vi "CA.vi"(0 "OUTPUT VARS":refnum<vi>, 1 "INPUT VARS":refnum<vi>, 2 "States":refnum<vi>, 3 "AlgStates":refnum<vi>, 4 "Processes":refnum<vi>, 5 "INP":refnum<vi>, 6 "PORTS":refnum<vi>) -> ()   [LabVIEW 2010]
panel:
  out "Здачения 2":string[](array[string])
  out "Типы 2":string[](array[string])
  out "Output:":string[](array[string])
  out "Value:":string[](array[string])
  out "Type:":string[](array[string])
  out "Input:":string[](array[string])
  out "Cluster":T1
  in  "algOutputMsgs":refnum<vi>
  in  "CA2GUI":refnum<vi>
  out "Output messages":T2(array[cluster])
  in  "OUTP":refnum<vi>
  out "Value":T3
  out "States of processes:":string[][](table)
  in  "OUT Ports Array":cluster{"Port":string, "Value":bool[]}[](array[cluster])
  in  "INP Ports Array":cluster{"Port\nPort":string, "Value":bool[]}[](array[cluster])
  # "Control algorithm"
  # "Global variables"
  # "Input ports values"
  # "Output ports values"
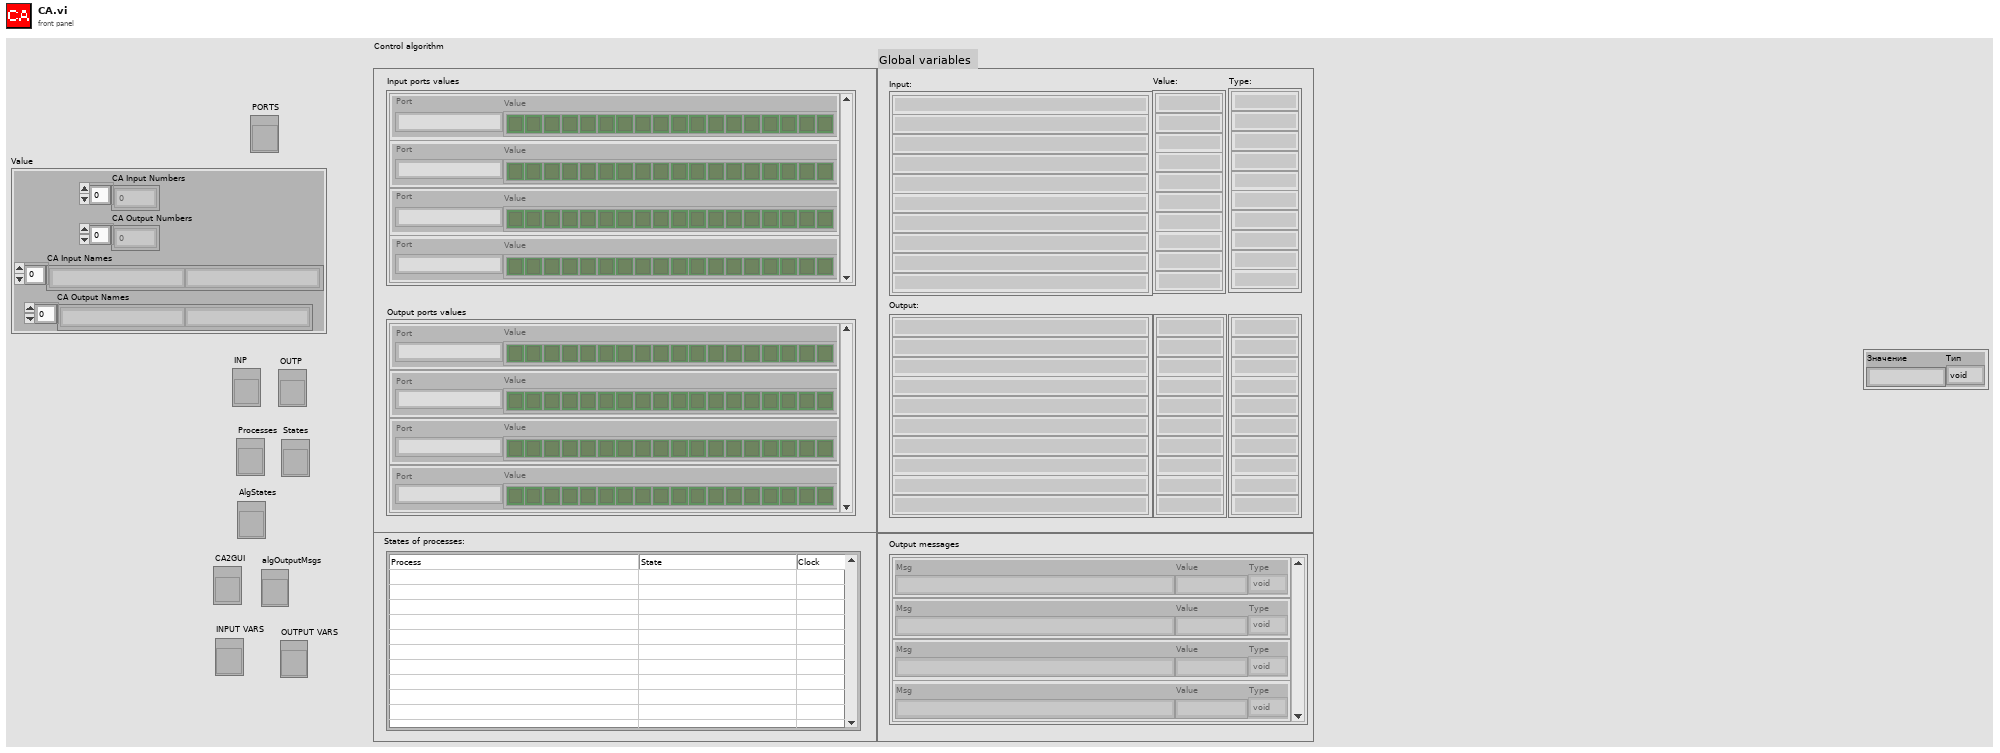
[diagram p1: front panel]
types:
  T1 = cluster{"Значение":string, "Тип":enum16{"void", "byte", "int", "float"}}
  T2 = cluster{"Msg":string, "Value":string, "Type":enum16{"void", "byte", "int", "float"}}[]
  T3 = cluster{"CA Input Numbers":i32[], "CA Output Numbers ":i32[], "CA Input Names":string[], "CA Output Names ":string[]}
  T4 = cluster{"Сообщение":string, "Значение":string, "Тип":enum16{"void", "byte", "int", "float"}}
  T5 = cluster{"Input varables names":string[], "Input varables type":string[], "Input varables ports":i32[], "Input varables bytes":i32[]}
  T6 = cluster{"Output varables names":string[], "Output varables type":string[], "Output varables ports":i32[], "Output varables bytes":i32[]}
  T7 = cluster{"Сообщение":string, "Значение":string, "Тип":enum16{"void", "byte", "int", "float"}}[]
  T8 = cluster{"MSG":i16, "param":i32, "Type":enum16{"void", "byte", "int", "float"}}[]
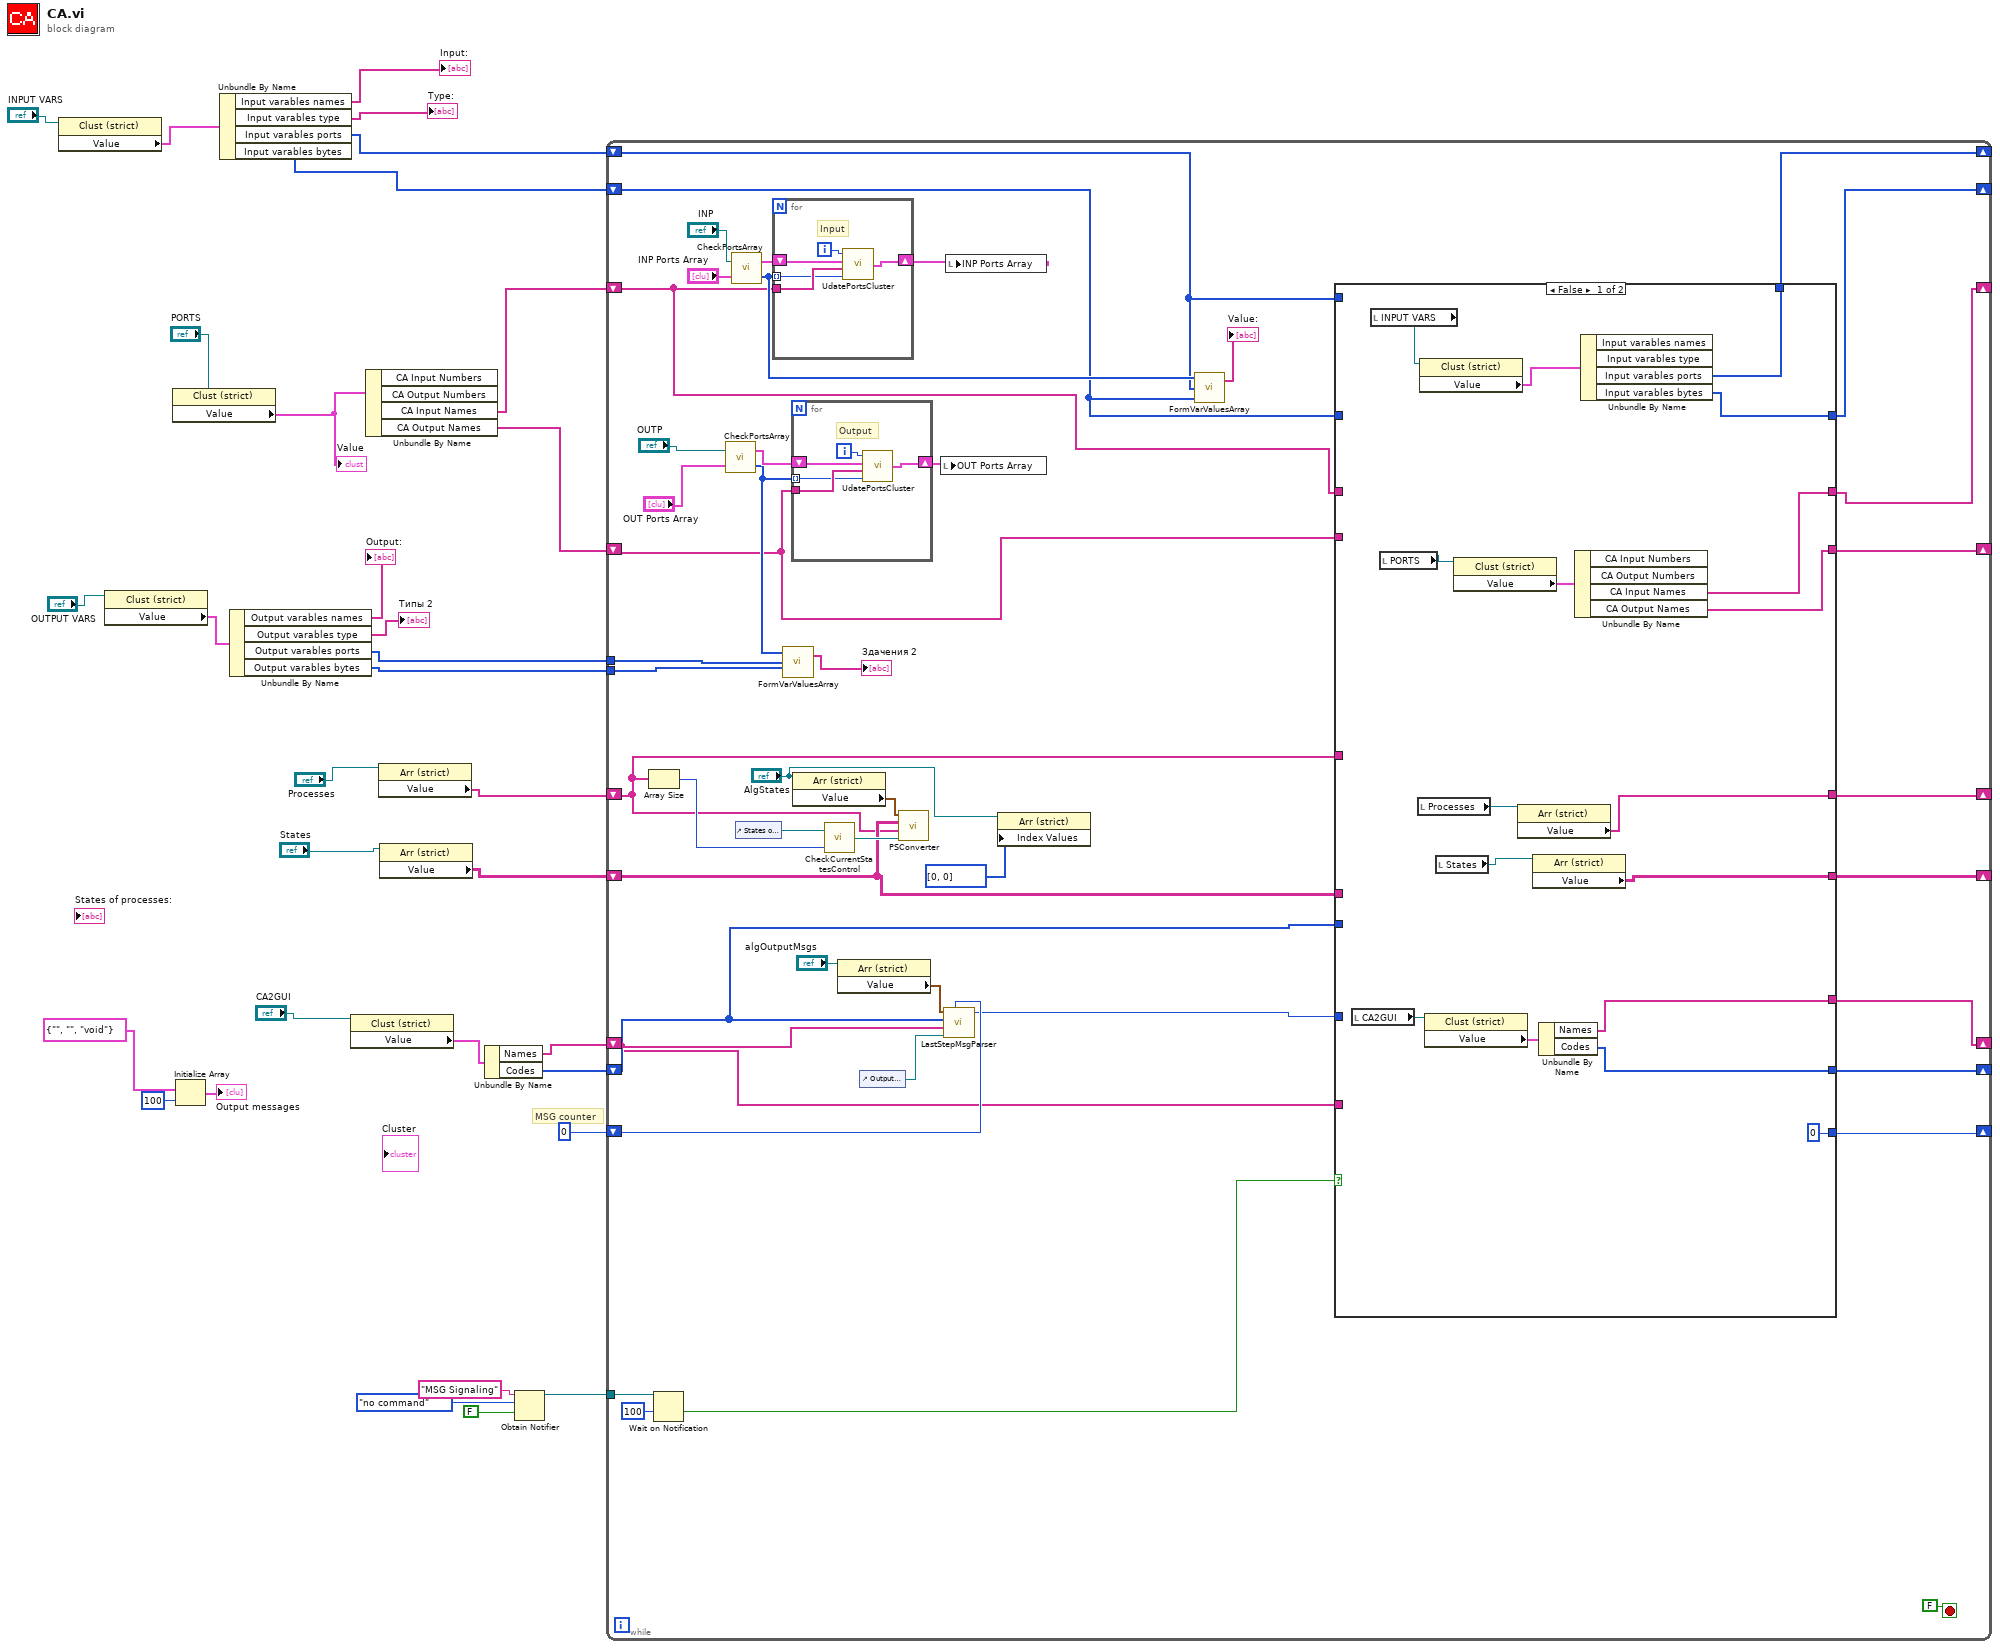
[diagram p0: block diagram]
diagram:
  # "MSG counter"
  n1 = property class="Clust (strict)"(reference="INPUT VARS") -> ("Value"=w16:T5)  [unwired: 1 in, 2 out]
  n2 = property class="Clust (strict)"(reference="OUTPUT VARS") -> ("Value"=w9:T6)  [unwired: 1 in, 2 out]
  n3 = property class="Clust (strict)"(reference="PORTS") -> ("Value"=w31:T3)  [unwired: 1 in, 2 out]
  "Value" <- w31
  n4 = Initialize Array(T4 {"Сообщение"="", "Значение"="", "Тип"=enum."void"} ("Cluster"), 100 ("dimension size")) -> (→"Output messages":T7)
  n5 = Unbundle By Name(w16) -> ("Input varables names"=→"Input:":string[], "Input varables type"=→"Type:":string[], "Input varables ports"=w15:i32[], "Input varables bytes"=w14:i32[])
  n6 = Unbundle By Name(w9) -> ("Output varables names"=→"Output:":string[], "Output varables type"=→"Типы 2":string[], "Output varables ports"=w6:i32[], "Output varables bytes"=w5:i32[])
  n7 = property class="Clust (strict)"(reference="CA2GUI") -> ("Value"=w24:cluster{"Names":string[], "Codes":i32[]})  [unwired: 1 in, 2 out]
  n8 = Unbundle By Name(w31) -> ("CA Input Names"=w30:string[], "CA Output Names"=w11:string[])  [unwired: 2 out]
  n9 = property class="Arr (strict)"(reference="Processes") -> ("Value"=w27:string[])  [unwired: 1 in, 2 out]
  n10 = property class="Arr (strict)"(reference="States") -> ("Value"=w26:string[][])  [unwired: 1 in, 2 out]
  n11 = Unbundle By Name(w24) -> ("Names"=w23:string[], "Codes"=w22:i32[])
  n12 = Obtain Notifier(name (unnamed)="MSG Signaling", notification data type=enum16{"no command", "refresh"}."no command", create if not found? (T)=FALSE) -> (notifier out=w1:refnum<notifier>)  [unwired: 1 in, 2 out]
  n13 = while {
    shift-right: [w51] -> _
    shift-left: 0 ("dimension size") -> [w61]
    tunnel: w6 -> [w58]
    tunnel: w5 -> [w57]
    tunnel: w1 -> [w54]
    shift-right: [w49] -> _
    shift-left: w22 -> [w50]
    shift-right: [w48] -> _
    shift-left: w23 -> [w47]
    shift-right: [w42] -> _
    shift-left: w26 -> [w45]
    shift-right: [w43] -> _
    shift-left: w27 -> [w44]
    shift-right: [w34] -> _
    shift-left: w14 -> [w40]
    shift-right: [w35] -> _
    shift-left: w15 -> [w41]
    shift-right: [w37] -> _
    shift-left: w11 -> [w38]
    shift-right: [w36] -> _
    shift-left: w30 -> [w39]
    stop <- FALSE ("stop") stop-if-true
    n14 = Array Size(array=w44) -> (size(s)=w46:i32)
    n15 = Wait on Notification(notifier=w54, timeout in ms (-1)=100) -> (timed out?=w53:bool)  [unwired: 2 in, 3 out]
    n16 = call "CheckPortsArray.vi"("INP Ports Array 2"="OUT Ports Array", "INP"="OUTP") -> ("Value"=w56:i8[], "INP Ports Array"=w72:cluster{"String":string, "Array 2":bool[]}[])
    n17 = call "CheckPortsArray.vi"("INP Ports Array 2"="INP Ports Array", "INP"="INP") -> ("Value"=w60:i8[], "INP Ports Array"=w76:cluster{"String":string, "Array 2":bool[]}[])
    n18 = control-ref of="States of processes:"() -> (w69:refnum<vi>)
    n19 = for {
      tunnel: w60 -> [w113] mode=indexing
      tunnel: w39 -> [w114]
      shift-right: [w110] -> w73
      shift-left: w76 -> [w111]
      i -> [w112]
      # "Input"
      n20 = call "UdatePortsCluster.vi"("Numeric 2"=w113, "Input Names"=w114, "Ports Array"=w111, "index"=w112) -> ("INP Ports Array 2"=w110:cluster{"String":string, "Array 2":bool[]}[])
    }
    n21 = call "FormVarValuesArray.vi"("varables bytes"=w57, "varables ports"=w58, "Ports"=w56) -> ("Values Array"=→"Здачения 2":string[])  [unwired: 1 in]
    n22 = for {
      tunnel: w56 -> [w108] mode=indexing
      tunnel: w38 -> [w109]
      shift-right: [w105] -> w71
      shift-left: w72 -> [w106]
      i -> [w107]
      # "Output"
      n23 = call "UdatePortsCluster.vi"("Numeric 2"=w108, "Input Names"=w109, "Ports Array"=w106, "index"=w107) -> ("INP Ports Array 2"=w105:cluster{"String":string, "Array 2":bool[]}[])
    }
    n24 = property class="Arr (strict)"(reference="AlgStates") -> ("Value"=w70:cluster{"TimeInState":u16, "cur_state":i8}[])  [unwired: 1 in, 2 out]
    n25 = call "CheckCurrentStatesControl.vi"("Processes"=w46, "Inp reference"=w69) -> ("Out Refnum"=w68:refnum<vi>)
    n26 = property class="Arr (strict)"(reference="algOutputMsgs") -> ("Value"=w63:T8)  [unwired: 1 in, 2 out]
    n27 = control-ref of="Output messages"() -> (w62:refnum<vi>)
    n28 = call "PSConverter.vi"("Current States 2"=w68, "PROC"=w44, "STATES"=w45, "Input claster"=w70) -> ()  [unwired: 1 out]
    n29 = local write "OUT Ports Array"(w71) -> ()
    n30 = call "LastStepMsgParser.vi"("Arr Refnum"=w62, "Out MSG Names"=w47, "old msg counter"=w61, "Codes"=w50, "Msg Array"=w63) -> ("current msg counter"=w52:i32)  [unwired: 4 in, 1 out]
    n31 = local write "INP Ports Array"(w73) -> ()
    n32 = property class="Arr (strict)"(reference="AlgStates", "Index Values"=u32[] [0, 0]) -> ()  [unwired: 1 in, 2 out]
    n33 = call "FormVarValuesArray.vi"("varables bytes"=w40, "varables ports"=w41, "Ports"=w60) -> ("Values Array"=→"Value:":string[])  [unwired: 1 in]
    n34 = case shown="False" w53 {
      tunnel: w52 -> [_ w102]
      tunnel: [0 ("current msg counter") w102] -> w51
      tunnel: w50 -> [_ w104]
      tunnel: [w91 w104] -> w49
      tunnel: [w92 w103] -> w48
      tunnel: w47 -> [_ w103]
      tunnel: w45 -> [_ w100]
      tunnel: w44 -> [_ w101]
      tunnel: [w89 w101] -> w43
      tunnel: [w87 w100] -> w42
      tunnel: w38 -> [_ w99]
      tunnel: w41 -> [_ w97]
      tunnel: w40 -> [_ w96]
      tunnel: w39 -> [_ w98]
      tunnel: [w84 w99] -> w37
      tunnel: [w83 w98] -> w36
      tunnel: [w80 w97] -> w35
      tunnel: [w79 w96] -> w34
      frame False {
        n35 = local read "CA2GUI"() -> (w94:refnum<vi>)
        n36 = local read "INPUT VARS"() -> (w81:refnum<vi>)
        n37 = local read "PORTS"() -> (w85:refnum<vi>)
        n38 = local read "Processes"() -> (w90:refnum<vi>)
        n39 = property class="Clust (strict)"(reference=w81) -> ("Value"=w82:T5)  [unwired: 1 in, 2 out]
        n40 = property class="Clust (strict)"(reference=w94) -> ("Value"=w93:cluster{"Names":string[], "Codes":i32[]})  [unwired: 1 in, 2 out]
        n41 = local read "States"() -> (w88:refnum<vi>)
        n42 = property class="Clust (strict)"(reference=w85) -> ("Value"=w86:T3)  [unwired: 1 in, 2 out]
        n43 = property class="Arr (strict)"(reference=w90) -> ("Value"=w89:string[])  [unwired: 1 in, 2 out]
        n44 = property class="Arr (strict)"(reference=w88) -> ("Value"=w87:string[][])  [unwired: 1 in, 2 out]
        n45 = Unbundle By Name(w93) -> ("Names"=w92:string[], "Codes"=w91:i32[])
        n46 = Unbundle By Name(w86) -> ("CA Input Names"=w83:string[], "CA Output Names"=w84:string[])  [unwired: 2 out]
        n47 = Unbundle By Name(w82) -> ("Input varables ports"=w80:i32[], "Input varables bytes"=w79:i32[])  [unwired: 2 out]
      }
      frame True {
      }
    }
  }
